vi "CameraGetData.vi"(8 "error in (no error)":errorcluster, 10 "keep open?":bool, 11 "AndorSDK2 in":refnum<class "Andor3.lvclass">) -> (0 "error out":errorcluster, 2 "image_data":u16[][][](array[numeric]), 3 "AndorSDK2 out":refnum<class "Andor3.lvclass">)   [LabVIEW 2010, in "Andor3.lvclass"]
uses:
  <userlib>/BIAS2/classes/Andor3/Andor3.lvclass
  <userlib>/BIAS2/classes/Andor3/Andor3.lvclass/Andor3.ctl
  <userlib>/atcoreA/atcoreA.lvlib
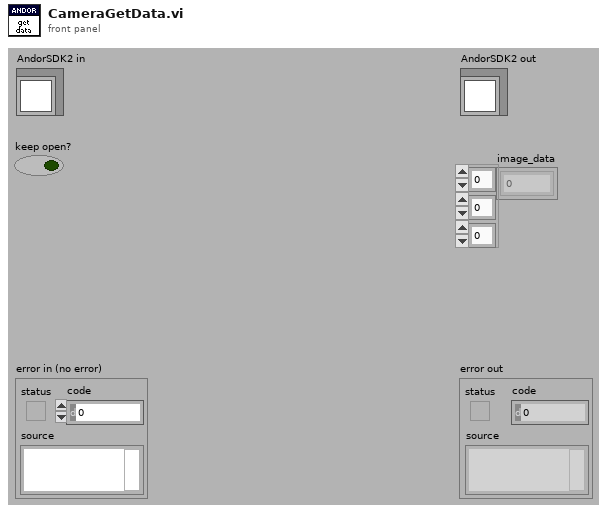
[diagram p1: front panel]
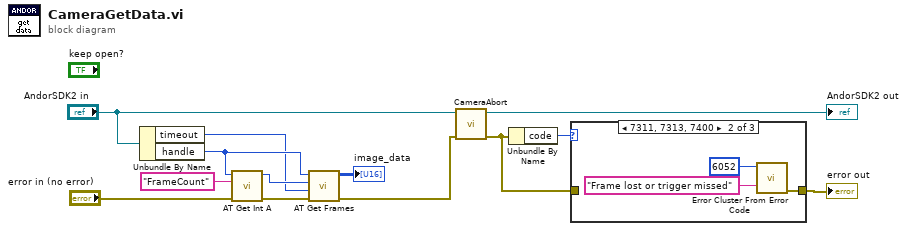
[diagram p0: block diagram]
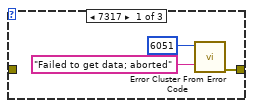
[diagram p2: hidden frame]
diagram:
  n1 = Unbundle By Name("AndorSDK2 in") -> ("timeout"=w1:u32, "handle"=w6:i32)
  n2 = call <userlib>:"AT Get Int A.vi"("error in (no error)"="error in (no error)", "Feature"="FrameCount", "Hndl"=w6) -> ("error out"=w5:errorcluster, "Value"=w7:i64)  [unwired: 7 in]
  n3 = call <userlib>:"AT Get Frames.vi"("error in (no error)"=w5, "timeout (ms)"=w1, "frames"=w7, "Hndl"=w6) -> ("error out"=w2:errorcluster, "data"=→"image_data":u16[][][])  [unwired: 2 in]
  n4 = call-dynamic "CameraAbort.vi"("error in"=w2, "AndorSDK3 in"="AndorSDK2 in") -> ("error out"=w10:errorcluster, "AndorSDK3 out"=→"AndorSDK2 out":refnum<class "Andor3.lvclass">)  [unwired: 8 in]
  n5 = Unbundle By Name(w10) -> ("code"=w11:i32)
  n6 = case shown="7311, 7313, 7400" w11 {
    tunnel: [w14 w17 w20] -> w9
    tunnel: w10 -> [_ _ w20]
    frame 7317 {
      n7 = call <vilib>:"Error Cluster From Error Code.vi"("error message (\"\")"="Failed to get data; aborted" ("error message (\"\")"), "error code (0)"=6051) -> ("error out"=w14:errorcluster)  [unwired: 7 in]
    }
    frame 7311, 7313, 7400 {
      n8 = call <vilib>:"Error Cluster From Error Code.vi"("error message (\"\")"="Frame lost or trigger missed" ("error message (\"\")"), "error code (0)"=6052) -> ("error out"=w17:errorcluster)  [unwired: 7 in]
    }
    frame Default {
    }
  }
  "error out" <- w9
